vi "Publish.vi"(8 "error in (no error)":errorcluster, 10 "PublishRequest":refnum<class "PublishRequest.lvclass">, 11 "Mediator in":refnum<class "Mediator.lvclass">) -> (0 "error out":errorcluster, 3 "Mediator out":refnum<class "Mediator.lvclass">)   [LabVIEW 2017, in "Mediator.lvlib" / "Mediator.lvclass"]
doc: "<License>\nCopyright © 2017 Composed Systems, LLC | All rights reserved\nwww.composed.io\n\nAuthor: Ethan Stern <ethan.stern@composed.io>\n\nThis software is provided \"AS IS\" WITHOUT WARRANTIES, either express or implied, AND IS FOR EDUCATIONAL PURPOSES ONLY.\n</License>"
uses:
  Mediator.lvclass
  IMediator/PublishRequest/PublishRequest.lvclass
  Mediator.lvclass/Mediator.ctl
  IMediator/PublishRequest/PublishRequest.lvclass/PublishRequest.ctl
  TopicLookupTable/TopicLookupTable.lvclass/TopicLookupTable.ctl
  Topic Messages/Notify Subscribers Msg/Notify Subscribers Msg.lvclass/Notify Subscribers Msg.ctl
  <vilib>/ActorFramework/Message Enqueuer/Message Enqueuer.lvclass/Message Enqueuer.ctl
  <vilib>/ActorFramework/Message Enqueuer/Enqueue.vi
  Topic Messages/Notify Subscribers Msg/Notify Subscribers Msg.lvclass
  C:/Program Files (x86)/National Instruments/LabVIEW 2017/vi.lib/ActorFramework/Message/Message.lvclass
  gpm_packages/@cs/variant/Source/Format Type String.vi
  <vilib>/ActorFramework/Message Priority Queue/Priority Enqueue.vi
  <vilib>/ActorFramework/Message Enqueuer/Message Enqueuer.lvclass
  TopicLookupTable/TopicLookupTable.lvclass
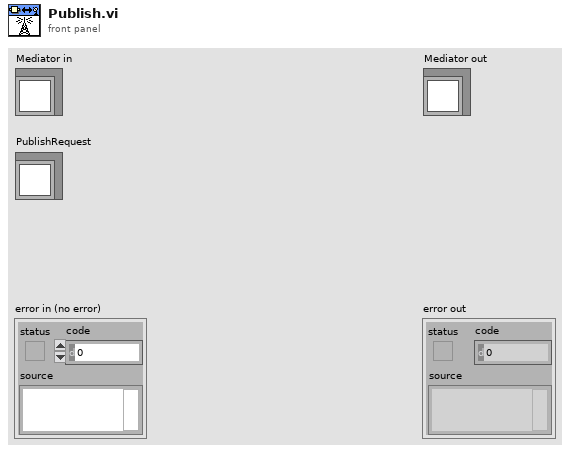
[diagram p1: front panel]
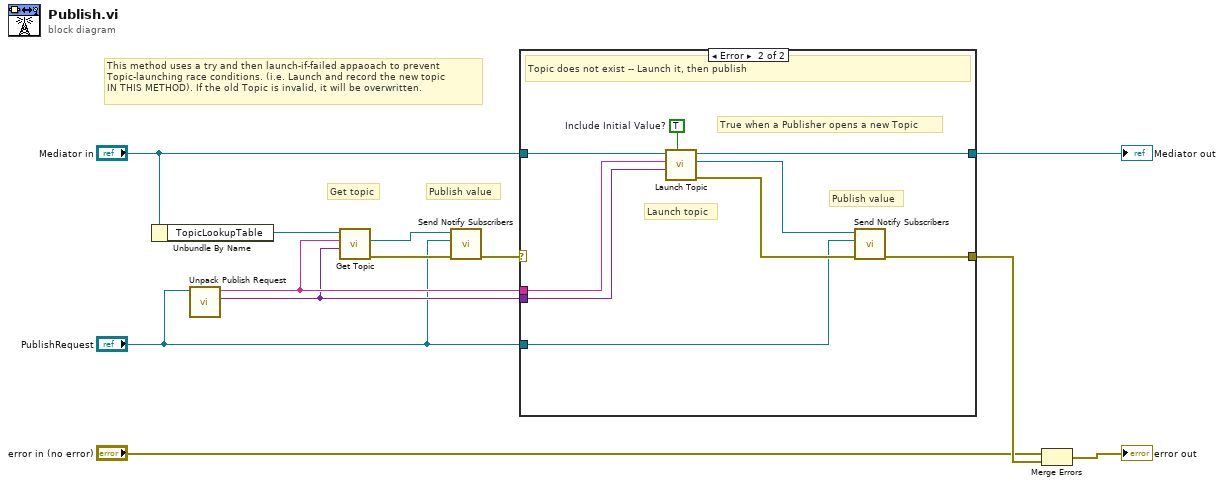
[diagram p0: block diagram]
diagram:
  # "This method uses a try and then launch-if-failed appaoach to prevent\nTopic-launching race conditions. (i.e. Launch and record the new topic\nIN THIS METHOD). If the old Topic is invalid, it will be overwritten."
  # "Publish value"
  # "Get topic"
  n1 = Unbundle By Name("Mediator in") -> ("TopicLookupTable"=w4:refnum<data-value>)
  n2 = call "Unpack Publish Request.vi"("PublishRequest In"="PublishRequest") -> ("Value"=w2:variant, "Datum Name"=w3:string)  [unwired: 7 in, 2 out]
  n3 = call "Get Topic.vi"("Topic Type"=w2, "Topic Name"=w3, "TopicLookupTable"=w4) -> ("error out"=w9:errorcluster, "Topic Enqueuer"=w12:refnum<class "Message Enqueuer.lvclass">)  [unwired: 6 in, 1 out]
  n4 = call "Send Notify Subscribers.vi"("error in (no error)"=w9, "PublishRequest"="PublishRequest", "Message Enqueuer"=w12) -> ("error out"=w11:errorcluster)  [unwired: 7 in, 1 out]
  n5 = case shown="Error" w11 {
    selector: w11 -> [w13 _]
    tunnel: "Mediator in" -> [w14 w23]
    tunnel: [w14 w21] -> w7
    tunnel: w3 -> [_ w19]
    tunnel: w2 -> [_ w18]
    tunnel: [w13 w22] -> w10
    tunnel: "PublishRequest" -> [_ w15]
    frame No Error {
      # "Topic exists -- Publish OK"
    }
    frame Error {
      w16 = TRUE  # Include Initial Value?
      # "True when a Publisher opens a new Topic"
      # "Launch topic"
      # "Publish value"
      # "Topic does not exist -- Launch it, then publish"
      n6 = call "Launch Topic.vi"("Include Initial Value? (F)"=w16, "Type"=w18, "Datum Name"=w19, "Mediator in"=w23) -> ("error out"=w17:errorcluster, "New Topic Enqueuer"=w20:refnum<class "Message Enqueuer.lvclass">, "Mediator out"=w21:refnum<class "Mediator.lvclass">)  [unwired: 5 in]
      n7 = call "Send Notify Subscribers.vi"("error in (no error)"=w17, "PublishRequest"=w15, "Message Enqueuer"=w20) -> ("error out"=w22:errorcluster)  [unwired: 7 in, 1 out]
    }
  }
  "Mediator out" <- w7
  n8 = Merge Errors("error in (no error)", w10) -> (→"error out":errorcluster)
